vi "Mechanum Convert.vi"(9 "Axes[1]":dbl, 10 "Axes[0]":dbl, 11 "Axes[2]":dbl) -> (0 "BackLeft":dbl, 1 "FrontLeft":dbl, 2 "BackRight":dbl, 3 "FrontRight":dbl)   [LabVIEW 2016]
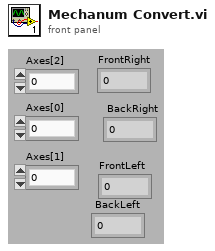
[diagram p1: front panel]
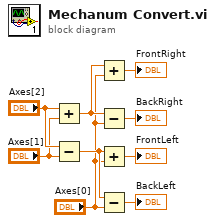
[diagram p0: block diagram]
diagram:
  n1 = Add(x="Axes[2]", y="Axes[1]") -> (x+y=w8:dbl)
  n2 = Subtract(x="Axes[2]", y="Axes[1]") -> (x-y=w9:dbl)
  n3 = Add(x=w8, y="Axes[0]") -> (x+y=→"FrontRight":dbl)
  n4 = Subtract(x=w8, y="Axes[0]") -> (x-y=→"BackRight":dbl)
  n5 = Add(x=w9, y="Axes[0]") -> (x+y=→"FrontLeft":dbl)
  n6 = Subtract(x=w9, y="Axes[0]") -> (x-y=→"BackLeft":dbl)
